vi "Anritsu VNA Sort Measurements.vi"(7 "Anritsu VNA":T6, 8 "error in (no error)":errorcluster, 9 "Auto Select":bool, 10 "Parameters to Measure":T1[](array[typedef]) {"Channel" min=1 max=99 step=1; "Parameter"."Stimulus Port" min=1 step=1; "Parameter"."Response Port" min=1 step=1}, 11 "VISA Resource Name":refnum<visa-resource-name>) -> (0 "error out":errorcluster {"code" format="%.0x"}, 1 "Channels Used":i8[](array[numeric]), 2 "Sorted Measurements":cluster{"Measurements":T5[]}[](array[cluster]) {"Measurements"."Traces"."Parameter"."Stimulus Port" min=1 step=1; "Measurements"."Traces"."Parameter"."Response Port" min=1 step=1}, 3 "dup VISA Resource Name":refnum<visa-resource-name>, 4 "Sorted Parameters to Measure":T1[](array[typedef]) {"Channel" min=1 max=99 step=1; "Parameter"."Stimulus Port" min=1 step=1; "Parameter"."Response Port" min=1 step=1}, 5 "Removed Parameters":T1[](array[typedef]) {"Channel" min=1 max=99 step=1; "Parameter"."Stimulus Port" min=1 step=1; "Parameter"."Response Port" min=1 step=1}, 6 "Measurements Removed?":bool)   [LabVIEW 2011]
uses:
  tests/S Parameter/TypeDefs/SP Parameter to Measure.ctl
  tests/S Parameter/TypeDefs/SP Parameter.ctl
  tests/S Parameter/TypeDefs/SP Calibration State.ctl
  tests/S Parameter/TypeDefs/SP Measurement Format.ctl
  TypeDefs/Anritsu VNA Instrument Info.ctl
  Agilent/TypeDefs/Agilent VNA Measurements.ctl
  Summitek/Win32/Miscellaneous/Add to Array if Not Present (I32).vi
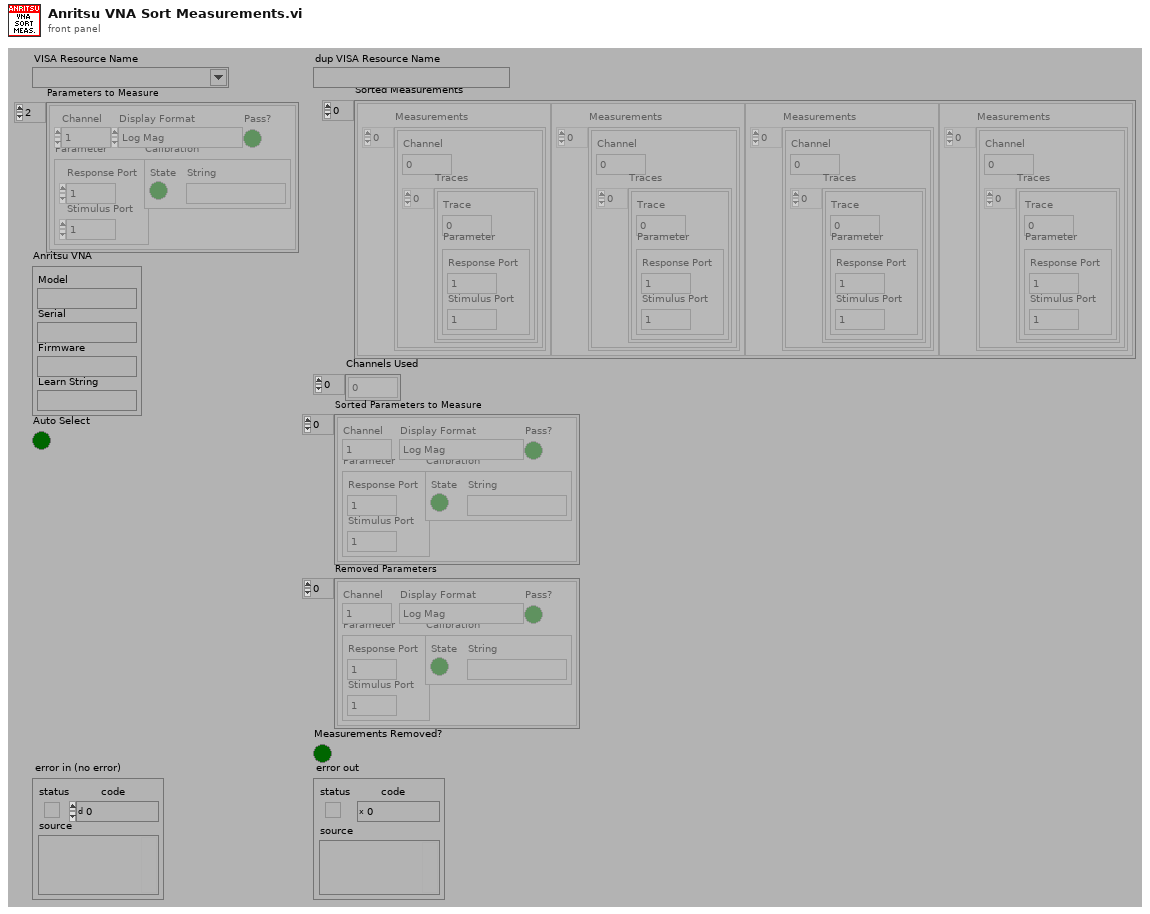
[diagram p1: front panel]
types:
  T1 = typedef "SP Parameter to Measure.ctl" = cluster{"Channel":i8, "Parameter":T2, "Calibration":T3, "Display Format":T4, "Pass?":bool}
  T2 = typedef "SP Parameter.ctl" = cluster{"Stimulus Port":i8, "Response Port":i8}
  T3 = typedef "SP Calibration State.ctl" = cluster{"State":bool, "String":string}
  T4 = typedef "SP Measurement Format.ctl" = enum32{"Log Mag", "Phase", "Delay", "Smith (R+jX)", "Polar (Re/Im)", "Linear Mag", "SWR", "Real", "Imaginary", "Smith (Lin/Phase)", "Smith (Log/Phase)", "Smith (Real/Imag)", "Smith (G+jB)", "Polar (Lin/Phase)", "Polar (Log/Phase)", "Expanded Phase", "Positive Phase", "Inverted Smith", "Unwrapped Phase", "Power Out", "Power In", "Linear Mag/Phase", "Log Mag/Phase", "Real/Imaginary"}
  T5 = typedef "Agilent VNA Measurements.ctl" = cluster{"Channel":i8, "Traces":cluster{"Trace":i8, "Parameter":T2}[]}
  T6 = typedef "Anritsu VNA Instrument Info.ctl" = cluster{"Model":string, "Serial":string, "Firmware":string, "Learn String":string}
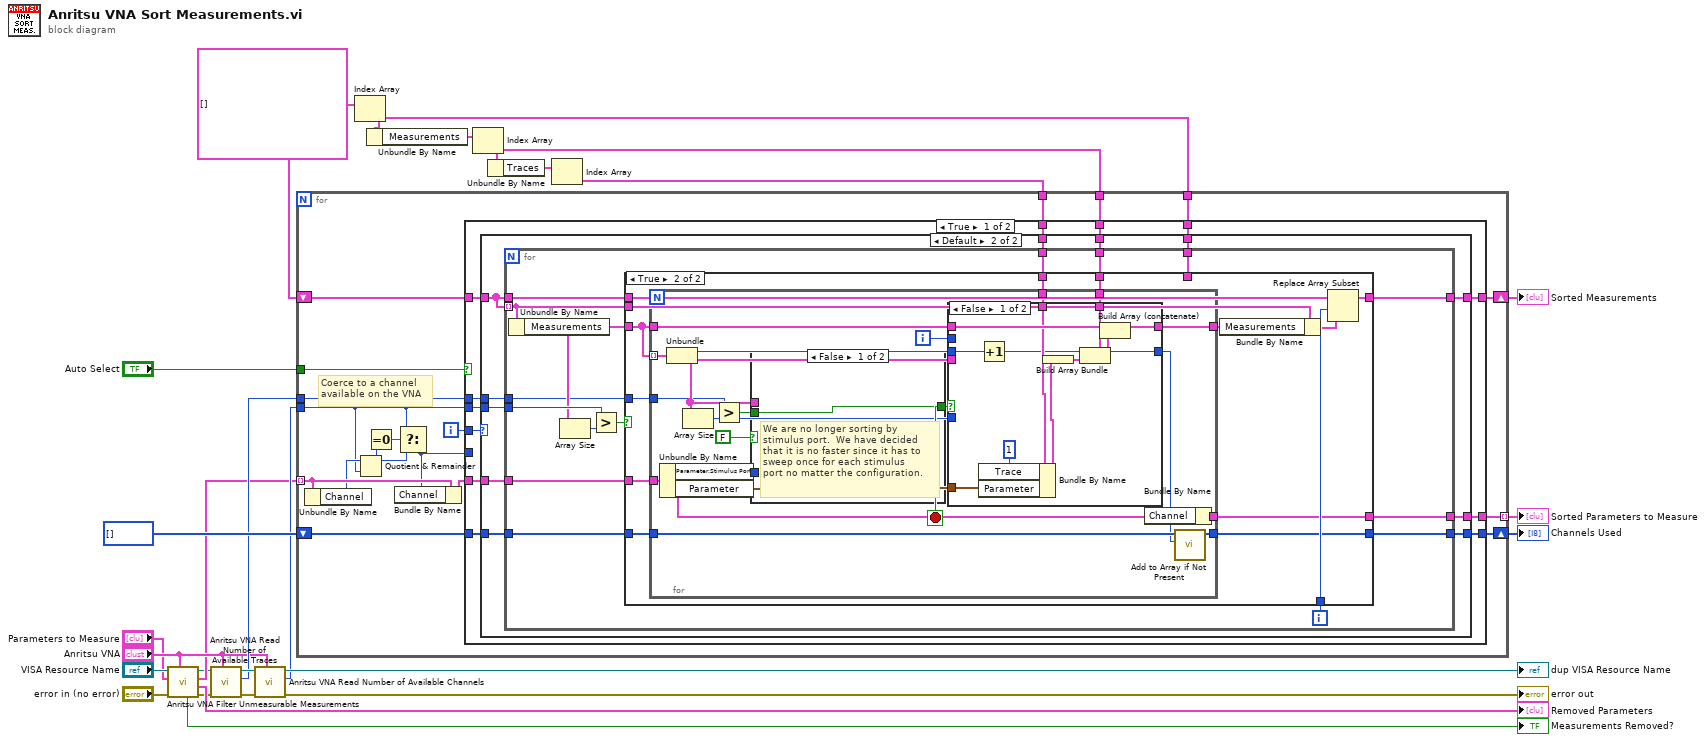
[diagram p0: block diagram]
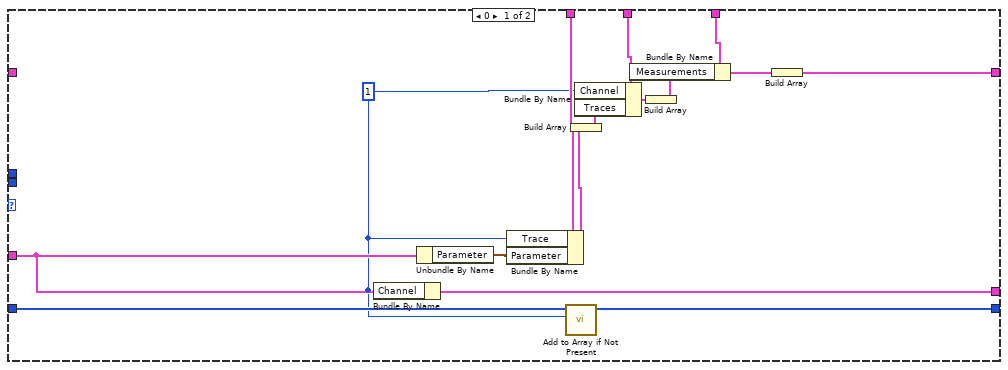
[diagram p2: hidden frame]
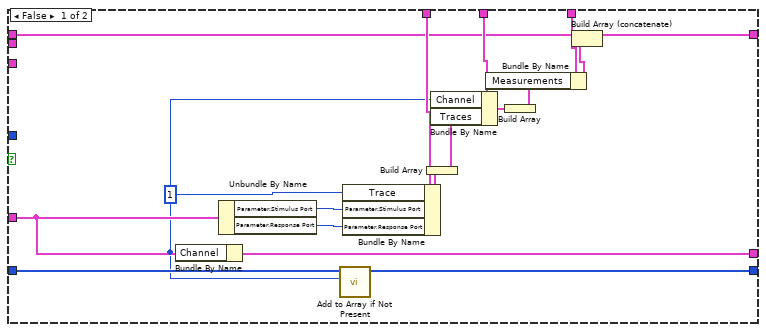
[diagram p3: hidden frame]
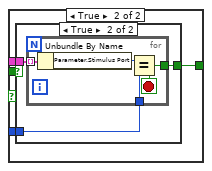
[diagram p4: hidden frame]
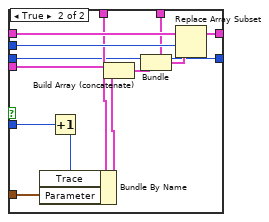
[diagram p6: hidden frame]
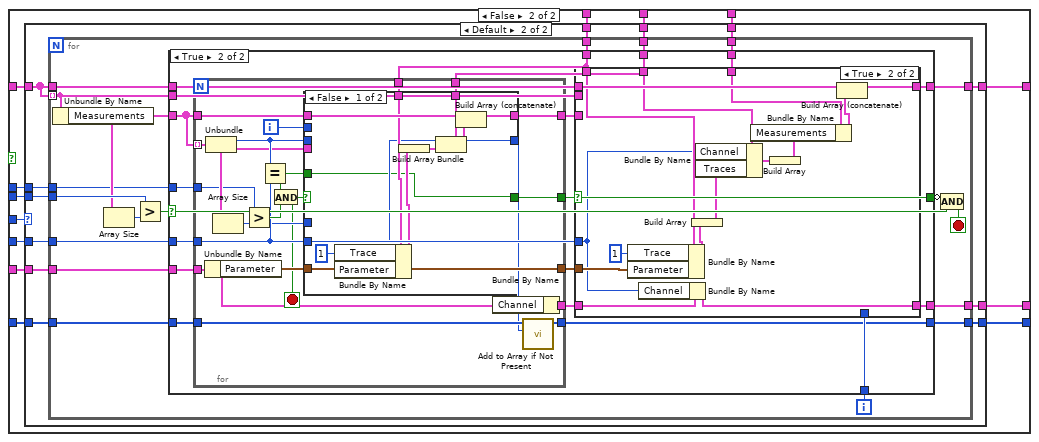
[diagram p7: hidden frame]
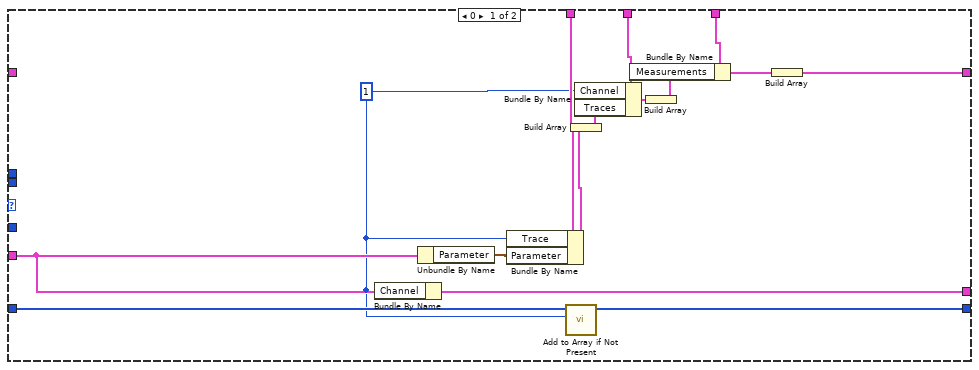
[diagram p8: hidden frame]
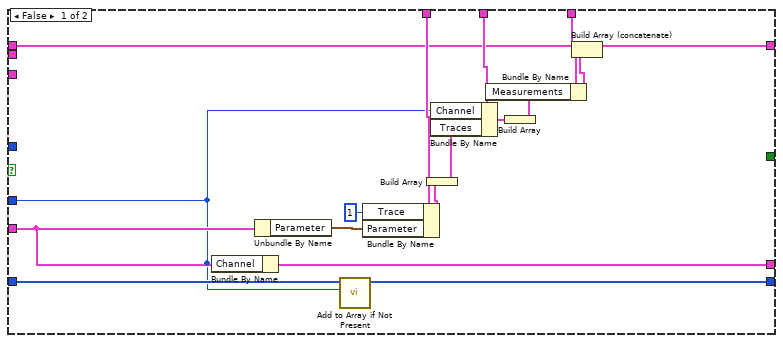
[diagram p9: hidden frame]
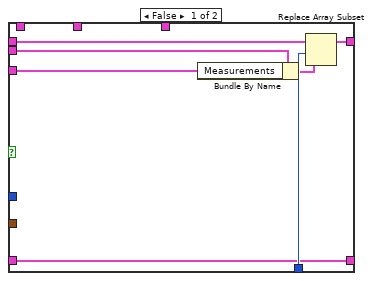
[diagram p10: hidden frame]
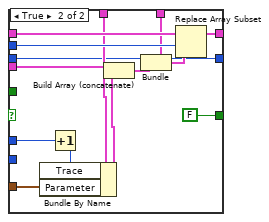
[diagram p11: hidden frame]
diagram:
  w21 = cluster{"Measurements":T5[]}[] [] ("Sorted Measurements")
  n1 = call "Anritsu VNA Filter Unmeasurable Measurements.vi"("Anritsu VNA"="Anritsu VNA", "error in (no error)"="error in (no error)", "Parameters to Measure"="Parameters to Measure", "VISA Resource Name"="VISA Resource Name") -> ("error out"=w3:errorcluster, "Removed Parameters"=→"Removed Parameters":T1[], "Filtered Parameters to Measure"=w6:T1[], "dup VISA Resource Name"=w2:refnum<visa-resource-name>, "Measurements Removed?"=→"Measurements Removed?":bool)  [unwired: 3 out]
  n2 = call "Anritsu VNA Read Number of Available Traces.vi"("Anritsu VNA"="Anritsu VNA", "error in (no error)"=w3, "VISA Resource Name"=w2) -> ("error out"=w13:errorcluster, "Number of Traces"=w11:i8, "dup VISA Resource Name"=w12:refnum<visa-resource-name>)  [unwired: 6 out]
  n3 = call "Anritsu VNA Read Number of Available Channels.vi"("Anritsu VNA"="Anritsu VNA", "error in (no error)"=w13, "VISA Resource Name"=w12) -> ("error out"=→"error out":errorcluster, "Number of Channels"=w14:i8, "dup VISA Resource Name"=→"dup VISA Resource Name":refnum<visa-resource-name>)  [unwired: 6 out]
  n4 = Index Array(array=w21) -> (element=w17:cluster{"Measurements":T5[]})  [unwired: 1 in]
  n5 = Unbundle By Name(w17) -> ("Measurements"=w23:T5[])
  n6 = Index Array(array=w23) -> (element=w18:T5)  [unwired: 1 in]
  n7 = Unbundle By Name(w18) -> ("Traces"=w20:cluster{"Trace":i8, "Parameter":T2}[])
  n8 = Index Array(array=w20) -> (element=w19:cluster{"Trace":i8, "Parameter":T2})  [unwired: 1 in]
  n9 = for {
    tunnel: w6 -> [w42] mode=indexing
    shift-right: [w32] -> w22
    shift-left: w21 -> [w43]
    tunnel: w14 -> [w37]
    tunnel: "Auto Select" -> [w35]
    tunnel: w19 -> [w34]
    tunnel: w18 -> [w33]
    tunnel: w17 -> [w31]
    shift-right: [w29] -> w15
    shift-left: i8[] [] -> [w30]
    tunnel: w11 -> [w28]
    tunnel: [w27] -> w1 mode=indexing
    i -> [w44]
    # "Coerce to a channel\navailable on the VNA"
    n10 = Unbundle By Name(w42) -> ("Channel"=w40:i8)
    n11 = Quotient & Remainder(x=w40, y=w37) -> (x-y*floor(x/y)=w36:i8)  [unwired: 1 out]
    n12 = Equal To 0?(x=w36) -> (x = 0?=w39:bool)
    n13 = Select(t=w37, s=w39, f=w36) -> (s? t:f=w38:i8)
    n14 = Bundle By Name(cluster=w42, "Channel"=w38) -> (w41:T1)
    n15 = case shown="True" w35 {
      tunnel: w44 -> [w50 w193]
      tunnel: w43 -> [w56 w199]
      tunnel: w41 -> [w55 w198]
      tunnel: w38 -> [_ w189]
      tunnel: w37 -> [w54 w197]
      tunnel: w34 -> [w53 w196]
      tunnel: w33 -> [w52 w195]
      tunnel: [w51 w194] -> w32
      tunnel: w31 -> [w49 w192]
      tunnel: w30 -> [w48 w191]
      tunnel: [w47 w190] -> w29
      tunnel: w28 -> [w46 w188]
      tunnel: [w45 w187] -> w27
      frame True {
        n16 = case shown="Default" w50 {
          tunnel: w56 -> [_ w77]
          tunnel: w55 -> [w59 w82]
          tunnel: w54 -> [_ w81]
          tunnel: w53 -> [w71 w80]
          tunnel: w52 -> [w69 w79]
          tunnel: [w62 w78] -> w51
          tunnel: w49 -> [w65 w76]
          tunnel: w48 -> [w61 w75]
          tunnel: [w60 w74] -> w47
          tunnel: w46 -> [_ w73]
          tunnel: [w58 w72] -> w45
          frame 0 {
            w57 = i8 1 ("Channel")
            n17 = Bundle By Name(cluster=w59, "Channel"=w57) -> (w58:T1)
            n18 = Unbundle By Name(w59) -> ("Parameter"=w70:T2)
            n19 = Bundle By Name(cluster=w71, "Trace"=w57, "Parameter"=w70) -> (w67:cluster{"Trace":i8, "Parameter":T2})
            n20 = call-poly "Add to Array if Not Present.vi"("I32"=w57, "I32 Array"=w61) -> ("New I32 Array"=w60:i32[])  [unwired: 3 out]
            n21 = Build Array(w67) -> (w66:cluster{"Trace":i8, "Parameter":T2}[])
            n22 = Bundle By Name(cluster=w69, "Channel"=w57, "Traces"=w66) -> (w68:T5)
            n23 = Build Array(w68) -> (w64:T5[])
            n24 = Bundle By Name(cluster=w65, "Measurements"=w64) -> (w63:cluster{"Measurements":T5[]})
            n25 = Build Array(w63) -> (w62:cluster{"Measurements":T5[]}[])
          }
          frame Default {
            n26 = for {
              tunnel: w77 -> [w91]
              tunnel: w82 -> [w98]
              tunnel: w81 -> [w94]
              tunnel: w80 -> [w97]
              tunnel: w79 -> [w96]
              tunnel: [w95] -> w78
              tunnel: w77 -> [w87] mode=indexing
              tunnel: w76 -> [w88]
              tunnel: w75 -> [w86]
              tunnel: [w85] -> w74
              tunnel: w73 -> [w84]
              tunnel: [w83] -> w72
              i -> [w90]
              n27 = Unbundle By Name(w87) -> ("Measurements"=w89:T5[])
              n28 = Array Size(array=w89) -> (size(s)=w93:i32)
              n29 = Greater?(x=w94, y=w93) -> (0:w92:bool)
              n30 = case shown="True" w92 {
                tunnel: w98 -> [w101 w129]
                tunnel: w97 -> [w112 w128]
                tunnel: w96 -> [w111 w127]
                tunnel: [w115 w124] -> w95
                tunnel: w89 -> [_ w126]
                tunnel: w91 -> [w108 w125]
                tunnel: w90 -> [_ w123]
                tunnel: w88 -> [w106 _]
                tunnel: w87 -> [_ w122]
                tunnel: w86 -> [w103 w119]
                tunnel: [w102 w118] -> w85
                tunnel: w84 -> [_ w117]
                tunnel: [w100 w116] -> w83
                frame False {
                  w99 = i8 1 ("Channel")
                  n31 = Bundle By Name(cluster=w101, "Channel"=w99) -> (w100:T1)
                  n32 = Unbundle By Name(w101) -> ("Parameter.Stimulus Port"=w114:i8, "Parameter.Response Port"=w113:i8)
                  n33 = call-poly "Add to Array if Not Present.vi"("I32"=w99, "I32 Array"=w103) -> ("New I32 Array"=w102:i32[])  [unwired: 3 out]
                  n34 = Bundle By Name(cluster=w112, "Trace"=w99, "Parameter.Stimulus Port"=w114, "Parameter.Response Port"=w113) -> (w110:cluster{"Trace":i8, "Parameter":T2})
                  n35 = Build Array(w110) -> (w109:cluster{"Trace":i8, "Parameter":T2}[])
                  n36 = Bundle By Name(cluster=w111, "Channel"=w99, "Traces"=w109) -> (w107:T5)
                  n37 = Build Array(w107) -> (w105:T5[])
                  n38 = Bundle By Name(cluster=w106, "Measurements"=w105) -> (w104:cluster{"Measurements":T5[]})
                  n39 = Build Array (concatenate)(w108, w104) -> (w115:cluster{"Measurements":T5[]}[])
                }
                frame True {
                  n40 = for {
                    tunnel: w126 -> [w145] mode=indexing
                    tunnel: w129 -> [w133]
                    tunnel: w126 -> [w149]
                    tunnel: [w146] -> w121
                    tunnel: w128 -> [w141]
                    tunnel: w127 -> [w139]
                    tunnel: w119 -> [w136]
                    tunnel: [w135] -> w118
                    tunnel: w117 -> [w134]
                    tunnel: [w131] -> w116
                    i -> [w148]
                    stop <- w144 stop-if-true
                    n41 = Unbundle By Name(w133) -> ("Parameter.Stimulus Port"=w137:i8, "Parameter"=w138:T2)
                    n42 = Unbundle(w145) -> ("Channel"=w142:i8, "Traces"=w143:cluster{"Trace":i8, "Parameter":T2}[])
                    n43 = Array Size(array=w143) -> (size(s)=w140:i32)
                    n44 = Greater?(x=w134, y=w140) -> (0:w147:bool)
                    n45 = case shown="False" FALSE {
                      tunnel: w147 -> [w150 w154]
                      tunnel: [w150 w153] -> w144
                      tunnel: w143 -> [_ w152]
                      tunnel: w137 -> [_ w151]
                      frame False {
                        # "We are no longer sorting by\nstimulus port.  We have decided\nthat it is no faster since it has to\nsweep once for each stimulus\nport no matter the configuration."
                      }
                      frame True {
                        n46 = case shown="True" w154 {
                          selector: w154 -> [w155 _]
                          tunnel: w152 -> [_ w158]
                          tunnel: [w155 w157] -> w153
                          tunnel: w151 -> [_ w156]
                          frame False {
                          }
                          frame True {
                            n47 = for {
                              tunnel: w158 -> [w162] mode=indexing
                              tunnel: [w160] -> w157
                              tunnel: w156 -> [w159]
                              stop <- w160 stop-if-true
                              n48 = Unbundle By Name(w162) -> ("Parameter.Stimulus Port"=w161:i8)
                              n49 = Equal?(x=w161, y=w159) -> (x = y?=w160:bool)
                            }
                          }
                        }
                      }
                    }
                    n50 = case shown="False" w144 {
                      tunnel: w143 -> [_ w182]
                      tunnel: w149 -> [w173 w186]
                      tunnel: w148 -> [_ w185]
                      tunnel: [w172 w184] -> w146
                      tunnel: w142 -> [w166 w174]
                      tunnel: w138 -> [w163 w180]
                      tunnel: w141 -> [w168 w181]
                      tunnel: w140 -> [_ w179]
                      tunnel: w139 -> [w169 w176]
                      tunnel: [w164 w174] -> w132
                      frame False {
                        n51 = Increment(x=w166) -> (x+1=w164:i8)
                        n52 = Bundle By Name(cluster=w168, "Trace"=i8 1, "Parameter"=w163) -> (w167:cluster{"Trace":i8, "Parameter":T2})
                        n53 = Build Array(w167) -> (w170:cluster{"Trace":i8, "Parameter":T2}[])
                        n54 = Bundle(cluster=w169, "Channel"=w164, "Traces"=w170) -> (w171:T5)
                        n55 = Build Array (concatenate)(w173, w171) -> (w172:T5[])
                      }
                      frame True {
                        n56 = Increment(x=w179) -> (x+1=w178:i32)
                        n57 = Bundle By Name(cluster=w181, "Trace"=w178, "Parameter"=w180) -> (w177:cluster{"Trace":i8, "Parameter":T2})
                        n58 = Build Array (concatenate)(w182, w177) -> (w175:cluster{"Trace":i8, "Parameter":T2}[])
                        n59 = Bundle(cluster=w176, "Channel"=w174, "Traces"=w175) -> (w183:T5)
                        n60 = Replace Array Subset(array=w186, new element=w183, index=w185) -> (w184:T5[])
                      }
                    }
                    n61 = Bundle By Name(cluster=w133, "Channel"=w132) -> (w131:T1)
                    n62 = call-poly "Add to Array if Not Present.vi"("I32"=w132, "I32 Array"=w136) -> ("New I32 Array"=w135:i32[])  [unwired: 3 out]
                  }
                  n63 = Bundle By Name(cluster=w122, "Measurements"=w121) -> (w120:cluster{"Measurements":T5[]})
                  n64 = Replace Array Subset(array=w125, new element=w120, index=w123) -> (w124:cluster{"Measurements":T5[]}[])
                }
              }
            }
          }
        }
      }
      frame False {
        n65 = case shown="Default" w193 {
          tunnel: w199 -> [_ w221]
          tunnel: w198 -> [w201 w226]
          tunnel: w197 -> [_ w225]
          tunnel: w196 -> [w214 w224]
          tunnel: w195 -> [w212 w223]
          tunnel: [w205 w222] -> w194
          tunnel: w192 -> [w208 w220]
          tunnel: w191 -> [w204 w219]
          tunnel: [w203 w218] -> w190
          tunnel: w189 -> [_ w217]
          tunnel: w188 -> [_ w216]
          tunnel: [w202 w215] -> w187
          frame 0 {
            w200 = i8 1 ("Channel")
            n66 = Bundle By Name(cluster=w201, "Channel"=w200) -> (w202:T1)
            n67 = Unbundle By Name(w201) -> ("Parameter"=w213:T2)
            n68 = Bundle By Name(cluster=w214, "Trace"=w200, "Parameter"=w213) -> (w210:cluster{"Trace":i8, "Parameter":T2})
            n69 = call-poly "Add to Array if Not Present.vi"("I32"=w200, "I32 Array"=w204) -> ("New I32 Array"=w203:i32[])  [unwired: 3 out]
            n70 = Build Array(w210) -> (w209:cluster{"Trace":i8, "Parameter":T2}[])
            n71 = Bundle By Name(cluster=w212, "Channel"=w200, "Traces"=w209) -> (w211:T5)
            n72 = Build Array(w211) -> (w207:T5[])
            n73 = Bundle By Name(cluster=w208, "Measurements"=w207) -> (w206:cluster{"Measurements":T5[]})
            n74 = Build Array(w206) -> (w205:cluster{"Measurements":T5[]}[])
          }
          frame Default {
            n75 = for {
              tunnel: w221 -> [w239]
              tunnel: w226 -> [w245]
              tunnel: w225 -> [w241]
              tunnel: w224 -> [w244]
              tunnel: w223 -> [w243]
              tunnel: [w242] -> w222
              tunnel: w221 -> [w235] mode=indexing
              tunnel: w220 -> [w236]
              tunnel: w219 -> [w234]
              tunnel: [w233] -> w218
              tunnel: w217 -> [w232]
              tunnel: w216 -> [w228]
              tunnel: [w227] -> w215
              i -> [w238]
              stop <- w229 stop-if-true
              n76 = Unbundle By Name(w235) -> ("Measurements"=w237:T5[])
              n77 = Array Size(array=w237) -> (size(s)=w240:i32)
              n78 = Greater?(x=w241, y=w240) -> (0:w230:bool)
              n79 = case shown="True" w230 {
                tunnel: w245 -> [w248 w280]
                tunnel: w244 -> [w260 w271]
                tunnel: w243 -> [w259 w270]
                tunnel: [w262 w277] -> w242
                tunnel: w237 -> [_ w279]
                tunnel: w239 -> [w256 w278]
                tunnel: w238 -> [_ w276]
                tunnel: w236 -> [w254 w267]
                tunnel: w235 -> [_ w275]
                tunnel: w234 -> [w251 w273]
                tunnel: [w250 w272] -> w233
                tunnel: w232 -> [w246 w268]
                tunnel: [_ w266] -> w231
                tunnel: w228 -> [_ w265]
                tunnel: [w247 w263] -> w227
                frame False {
                  n80 = Bundle By Name(cluster=w248, "Channel"=w246) -> (w247:T1)
                  n81 = Unbundle By Name(w248) -> ("Parameter"=w261:T2)
                  n82 = call-poly "Add to Array if Not Present.vi"("I32"=w246, "I32 Array"=w251) -> ("New I32 Array"=w250:i32[])  [unwired: 3 out]
                  n83 = Bundle By Name(cluster=w260, "Trace"=i8 1 ("Channel"), "Parameter"=w261) -> (w258:cluster{"Trace":i8, "Parameter":T2})
                  n84 = Build Array(w258) -> (w257:cluster{"Trace":i8, "Parameter":T2}[])
                  n85 = Bundle By Name(cluster=w259, "Channel"=w246, "Traces"=w257) -> (w255:T5)
                  n86 = Build Array(w255) -> (w253:T5[])
                  n87 = Bundle By Name(cluster=w254, "Measurements"=w253) -> (w252:cluster{"Measurements":T5[]})
                  n88 = Build Array (concatenate)(w256, w252) -> (w262:cluster{"Measurements":T5[]}[])
                }
                frame True {
                  n89 = for {
                    tunnel: w279 -> [w320] mode=indexing
                    tunnel: w280 -> [w305]
                    tunnel: w279 -> [w323]
                    tunnel: [w321] -> w274
                    tunnel: w271 -> [w319]
                    tunnel: w270 -> [w318]
                    tunnel: w273 -> [w317]
                    tunnel: [w316] -> w272
                    tunnel: w268 -> [w311]
                    tunnel: [w314] -> w269
                    tunnel: [w308] -> w266
                    tunnel: w265 -> [w306]
                    tunnel: [w303] -> w264
                    i -> [w322]
                    stop <- w309 stop-if-true
                    n90 = Unbundle By Name(w305) -> ("Parameter"=w314:T2)
                    n91 = Unbundle(w320) -> ("Channel"=w315:i8, "Traces"=w313:cluster{"Trace":i8, "Parameter":T2}[])
                    n92 = Array Size(array=w313) -> (size(s)=w310:i32)
                    n93 = Greater?(x=w306, y=w310) -> (0:w312:bool)
                    n94 = Equal?(x=w315, y=w311) -> (x = y?=w307:bool)
                    n95 = And(x=w307, y=w312) -> (x .and. y?=w309:bool)
                    n96 = case shown="False" w309 {
                      tunnel: w313 -> [_ w344]
                      tunnel: w323 -> [w334 w348]
                      tunnel: w322 -> [_ w347]
                      tunnel: [w333 w346] -> w321
                      tunnel: w315 -> [_ w338]
                      tunnel: w314 -> [w327 w342]
                      tunnel: w319 -> [w329 w343]
                      tunnel: w318 -> [w330 w340]
                      tunnel: [w325 w338] -> w304
                      tunnel: w311 -> [w325 _]
                      tunnel: w310 -> [_ w337]
                      tunnel: [w324 FALSE] -> w308
                      tunnel: w307 -> [w324 _]
                      frame False {
                        n97 = Bundle By Name(cluster=w329, "Trace"=i8 1, "Parameter"=w327) -> (w328:cluster{"Trace":i8, "Parameter":T2})
                        n98 = Build Array(w328) -> (w331:cluster{"Trace":i8, "Parameter":T2}[])
                        n99 = Bundle(cluster=w330, "Channel"=w325, "Traces"=w331) -> (w332:T5)
                        n100 = Build Array (concatenate)(w334, w332) -> (w333:T5[])
                      }
                      frame True {
                        n101 = Increment(x=w337) -> (x+1=w336:i32)
                        n102 = Bundle By Name(cluster=w343, "Trace"=w336, "Parameter"=w342) -> (w341:cluster{"Trace":i8, "Parameter":T2})
                        n103 = Build Array (concatenate)(w344, w341) -> (w339:cluster{"Trace":i8, "Parameter":T2}[])
                        n104 = Bundle(cluster=w340, "Channel"=w338, "Traces"=w339) -> (w345:T5)
                        n105 = Replace Array Subset(array=w348, new element=w345, index=w347) -> (w346:T5[])
                      }
                    }
                    n106 = Bundle By Name(cluster=w305, "Channel"=w304) -> (w303:T1)
                    n107 = call-poly "Add to Array if Not Present.vi"("I32"=w304, "I32 Array"=w317) -> ("New I32 Array"=w316:i32[])  [unwired: 3 out]
                  }
                  n108 = case shown="True" w266 {
                    tunnel: w278 -> [w287 w296]
                    tunnel: [w286 w295] -> w277
                    tunnel: w276 -> [w285 _]
                    tunnel: w275 -> [w284 _]
                    tunnel: w274 -> [w283 _]
                    tunnel: w271 -> [_ w294]
                    tunnel: w270 -> [_ w292]
                    tunnel: w269 -> [_ w293]
                    tunnel: w268 -> [_ w288]
                    tunnel: w267 -> [_ w291]
                    tunnel: w264 -> [w281 w290]
                    tunnel: [w281 w289] -> w263
                    frame False {
                      n109 = Bundle By Name(cluster=w284, "Measurements"=w283) -> (w282:cluster{"Measurements":T5[]})
                      n110 = Replace Array Subset(array=w287, new element=w282, index=w285) -> (w286:cluster{"Measurements":T5[]}[])
                    }
                    frame True {
                      n111 = Bundle By Name(cluster=w294, "Trace"=i8 1 ("Channel"), "Parameter"=w293) -> (w302:cluster{"Trace":i8, "Parameter":T2})
                      n112 = Bundle By Name(cluster=w290, "Channel"=w288) -> (w289:T1)
                      n113 = Build Array(w302) -> (w301:cluster{"Trace":i8, "Parameter":T2}[])
                      n114 = Bundle By Name(cluster=w292, "Channel"=w288, "Traces"=w301) -> (w300:T5)
                      n115 = Build Array(w300) -> (w299:T5[])
                      n116 = Bundle By Name(cluster=w291, "Measurements"=w299) -> (w298:cluster{"Measurements":T5[]})
                      n117 = Build Array (concatenate)(w296, w298) -> (w295:cluster{"Measurements":T5[]}[])
                    }
                  }
                }
              }
              n118 = Compound Arithmetic op=AND(invert w231, w230) -> (w229:bool)
            }
          }
        }
      }
    }
  }
  "Sorted Measurements" <- w22
  "Channels Used" <- w15
  "Sorted Parameters to Measure" <- w1
